vi "GetParent.vi"(0 "object in":refnum<class "Node.lvclass">, 5 "Error In":errorcluster) -> (14 "object out":refnum<class "Node.lvclass">, 15 "Parent":refnum<class "Element.lvclass">, 19 "Error Out":errorcluster)   [LabVIEW 2024, in "Node.lvclass"]
uses:
  <resource>/Framework/Providers/Open_GDS/ClassProviders/Provider_LvNativeClass/Templates/NativeBaseTemplate/NativeBaseTemplate.lvclass/NativeBaseTemplate.ctl
  Node.lvclass
  Node.lvclass/Node.ctl
  Element_interface/Element.lvclass
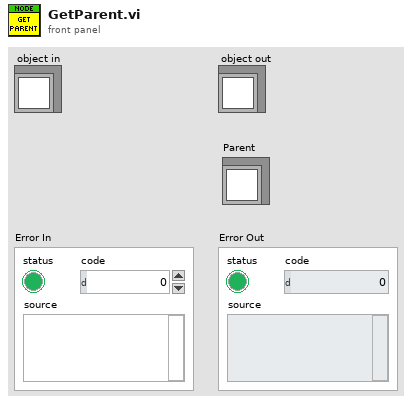
[diagram p1: front panel]
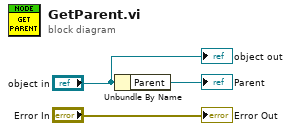
[diagram p0: block diagram]
diagram:
  n1 = Unbundle By Name("object in") -> ("Parent"=→"Parent":refnum<class "Element.lvclass">)
  "Error Out" <- "Error In"
  "object out" <- "object in"
